vi "Do Request.vi"(7 "Processing In":refnum<class "Processing.lvclass">, 11 "Submit in":refnum<class "Submit.lvclass">) -> (0 "error out":errorcluster, 5 "Processing":refnum<class "Processing.lvclass">)   [LabVIEW 2020, in "Summer of LabVIEW.lvlib" / "Submit.lvclass"]
uses:
  Submit.lvclass
  Submit.lvclass/Submit.ctl
  <vilib>/IlluminatedG/IG HTTP Server/HTTP Server/Processing/Processing.lvclass
  e66c75b8-1da6-49a6-8e93-b7de8044fac6.vi
  05b68bd3-c3cb-4105-86e0-25e66e7234fa.vi
  Challenge DB/Challenge DB.lvclass
  <vilib>/IlluminatedG/IG HTTP Utils/HTTP Utils/Request/Request.lvclass
  <vilib>/IlluminatedG/IG HTTP Utils/HTTP Utils/FormField/FormField.lvclass
  <vilib>/IlluminatedG/IG HTTP Utils/HTTP Utils/Response/Response.lvclass
  Challenge/Challenge.lvclass
  SOL User/SOL User.lvclass
  648c7329-21b3-4aca-ab96-64ccfe930613.vi
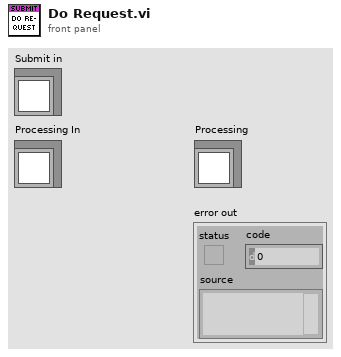
[diagram p1: front panel]
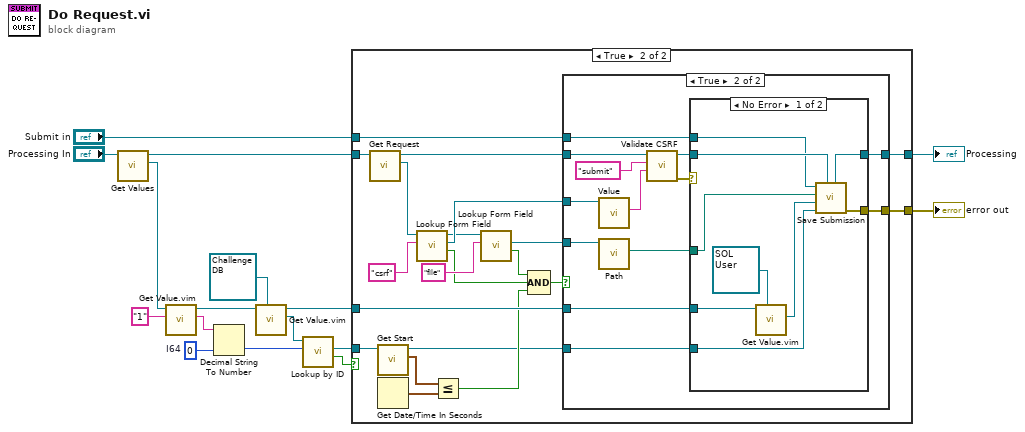
[diagram p0: block diagram]
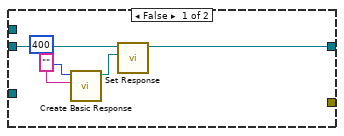
[diagram p3: hidden frame]
diagram:
  w5 = i64 0  # I64
  n1 = call <vilib>:"Get Values.vi"("Processing in"="Processing In") -> ("Values"=w15:refnum<class "Values.lvclass">, "Processing out"=w7:refnum<class "Processing.lvclass">)  [unwired: 9 in]
  n2 = call "Get Value.vim"("Name for Type"="1", "Arguments in"=w15) -> ("Value"=w6:string, "Arguments out"=w13:refnum<class "Values.lvclass">)  [unwired: 7 in, 1 out]
  n3 = Decimal String To Number(string=w6, default (0L)=w5) -> (number=w4:i64)  [unwired: 1 in, 1 out]
  n4 = call "Get Value.vim"("Type / Server / Service (String)"=refnum<class "Challenge DB.lvclass"> refnum ("SOL:Challenge DB.lvclass"), "Arguments in"=w13) -> ("Value"=w11:refnum<class "Challenge DB.lvclass">, "Arguments out"=w8:refnum<class "Values.lvclass">)  [unwired: 7 in, 1 out]
  n5 = call "Lookup by ID.vi"("ID"=w4, "Challenge DB in"=w11) -> ("Found?"=w10:bool, "Challenge"=w9:refnum<class "Challenge.lvclass">)  [unwired: 6 in, 2 out]
  n6 = case shown="True" w10 {
    tunnel: w9 -> [_ w23]
    tunnel: w8 -> [_ w28]
    tunnel: w7 -> [w17 w37]
    tunnel: [w17 w26] -> w3
    tunnel: [_ w25] -> w2
    tunnel: "Submit in" -> [_ w18]
    frame False {
    }
    frame True {
      n7 = call <vilib>:"Get Request.vi"("Processing in"=w37) -> ("Request"=w36:refnum<class "Request.lvclass">, "Processing out"=w27:refnum<class "Processing.lvclass">)  [unwired: 9 in]
      n8 = call "Get Start.vi"("Challenge in"=w23) -> ("Start"=w22:timestamp, "Challenge out"=w19:refnum<class "Challenge.lvclass">)  [unwired: 9 in]
      n9 = Get Date/Time In Seconds() -> (seconds since 1Jan1904=w21:timestamp)
      n10 = call <vilib>:"Lookup Form Field.vi"("Name"="csrf", "Request in"=w36) -> ("Exists"=w32:bool, "Field"=w29:refnum<class "FormField.lvclass">, "Request out"=w24:refnum<class "Request.lvclass">)  [unwired: 6 in, 1 out]
      n11 = Less Or Equal?(x=w22, y=w21) -> (x <= y?=w20:bool)
      n12 = call <vilib>:"Lookup Form Field.vi"("Name"="file", "Request in"=w24) -> ("Exists"=w33:bool, "Field"=w30:refnum<class "FormField.lvclass">)  [unwired: 6 in, 2 out]
      n13 = Compound Arithmetic op=AND(w33, w32, w20) -> (w31:bool)
      n14 = case shown="True" w31 {
        tunnel: w30 -> [_ w47]
        tunnel: w29 -> [_ w55]
        tunnel: w28 -> [_ w45]
        tunnel: w19 -> [_ w44]
        tunnel: w27 -> [w40 w54]
        tunnel: [w38 w49] -> w26
        tunnel: [_ w50] -> w25
        tunnel: w18 -> [_ w43]
        frame False {
          n15 = call <vilib>:"Create Basic Response.vi"("Payload"="", "Status Code"=u16 400) -> ("Response out"=w39:refnum<class "Response.lvclass">)  [unwired: 8 in, 1 out]
          n16 = call <vilib>:"Set Response.vi"("Response"=w39, "Processing in"=w40) -> ("Processing out"=w38:refnum<class "Processing.lvclass">)  [unwired: 9 in]
        }
        frame True {
          n17 = call <vilib>:"Value.vi"("FormField in"=w55) -> ("Value"=w48:string)  [unwired: 8 in, 2 out]
          n18 = call <vilib>:"Path.vi"("FormField in"=w47) -> ("Path"=w46:path)  [unwired: 8 in, 2 out]
          n19 = call <vilib>:"Validate CSRF.vi"("Token"=w48, "Token ID"="submit", "Processing in"=w54) -> ("error out"=w52:errorcluster, "Processing out"=w51:refnum<class "Processing.lvclass">)  [unwired: 7 in]
          n20 = case shown="No Error" w52 {
            selector: w52 -> [_ w66]
            tunnel: w51 -> [w57 w65]
            tunnel: [w59 w66] -> w50
            tunnel: [w58 w65] -> w49
            tunnel: w46 -> [w62 _]
            tunnel: w45 -> [w64 _]
            tunnel: w44 -> [w60 _]
            tunnel: w43 -> [w56 _]
            frame No Error {
              n21 = call "Get Value.vim"("Type / Server / Service (String)"=refnum<class "SOL User.lvclass"> refnum ("SOL:SOL User.lvclass"), "Arguments in"=w64) -> ("Value"=w61:refnum<class "SOL User.lvclass">)  [unwired: 7 in, 2 out]
              n22 = call "Save Submission.vi"("Processing in"=w57, "Challenge"=w60, "User"=w61, "File Path"=w62, "Submit"=w56) -> ("error out"=w59:errorcluster, "Processing out"=w58:refnum<class "Processing.lvclass">)  [unwired: 5 in]
            }
            frame Error {
            }
          }
        }
      }
    }
  }
  "error out" <- w2
  "Processing" <- w3
